vi "ad continu.vi"(0 "dev":i32, 1 "ad_os":i32, 2 "ad_range":i32, 3 "ch_first":i32, 4 "ch_last":i32, 5 "freq":i32, 6 "trig_sl":i32, 7 "error in (no error)":errorcluster caption="错误输入（无错误）", 8 "trig_pol":i32, 9 "clk_sl":i32, 10 "ext_clk_pol":i32, 11 "num":i32, 12 "databuf":sgl) -> (14 "databuf out":sgl, 20 "function return":i32, 27 "error out":errorcluster caption="错误输出")   [LabVIEW 2018, in "恒凯采集卡.lvlib"]
doc: "int ad_continu(int dev,int ad_os,int ad_range,int ch_first,int ch_last,int freq,int trig_sl,int trig_pol,int clk_sl,int ext_clk_pol,int num,float* databuf);"
uses:
  data/Usb_Daq_V52_32.dll
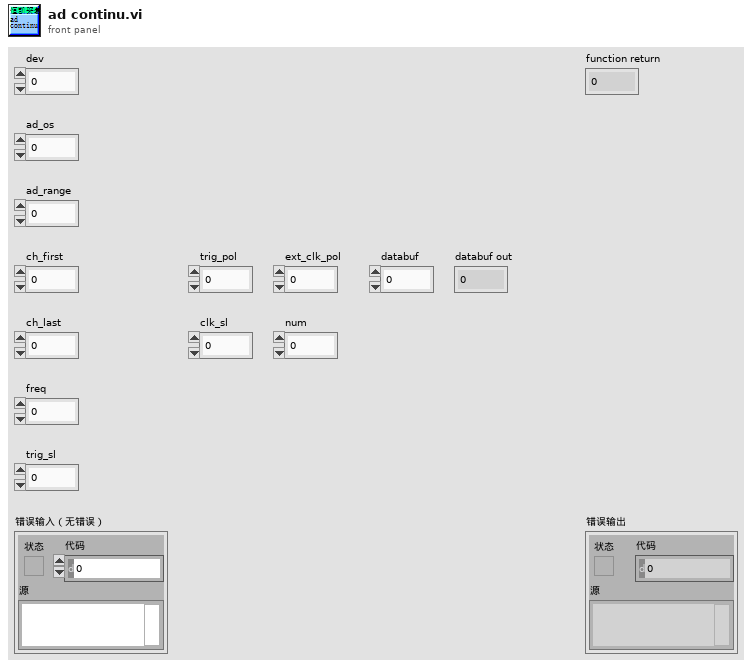
[diagram p1: front panel]
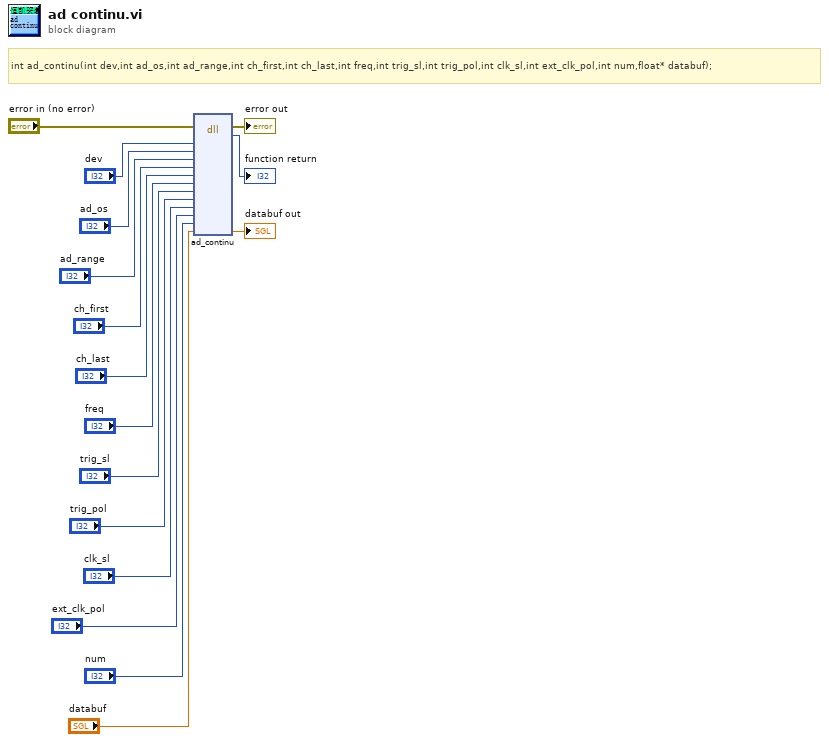
[diagram p0: block diagram]
diagram:
  # "int ad_continu(int dev,int ad_os,int ad_range,int ch_first,int ch_last,int freq,int trig_sl,int trig_pol,int clk_sl,int ext_clk_pol,int num,float* databuf);"
  n1 = dll-call lib="D:/ProgramFiles/NI/LabVIEW 2018/user.lib/Usb_Daq_V52_32/Usb_Daq_V52_32.*" fn="ad_continu"(error in="error in (no error)", "dev"="dev", "ad_os"="ad_os", "ad_range"="ad_range", "ch_first"="ch_first", "ch_last"="ch_last", "freq"="freq", "trig_sl"="trig_sl", "trig_pol"="trig_pol", "clk_sl"="clk_sl", "ext_clk_pol"="ext_clk_pol", "num"="num", "databuf"="databuf") -> (error out=→"error out":errorcluster, →"function return":i32, "databuf"=→"databuf out":sgl)  [unwired: 13 in, 1 out]
